vi "ACT_effective_setpoint.vi"(8 "error in (no error)":errorcluster, 11 "MD420 in":refnum<class "MD420.lvclass">) -> (0 "error out":errorcluster, 3 "MD420 out":refnum<class "MD420.lvclass">)   [LabVIEW 2022 SP3, in "MD420.lvclass"]
uses:
  MD420.lvclass
  SI_modules/SI656/SI656.lvclass
  SI_modules/SI657/SI657.lvclass
  MD420.lvclass/MD420.ctl
panel:
  in  "SI657.lvclass":refnum<class "SI657.lvclass">
  in  "SI656 in":refnum<class "SI656.lvclass">
  in  "PG SP-Grad":dbl
  in  "ACT-Ctrl ON (MD404)":dbl
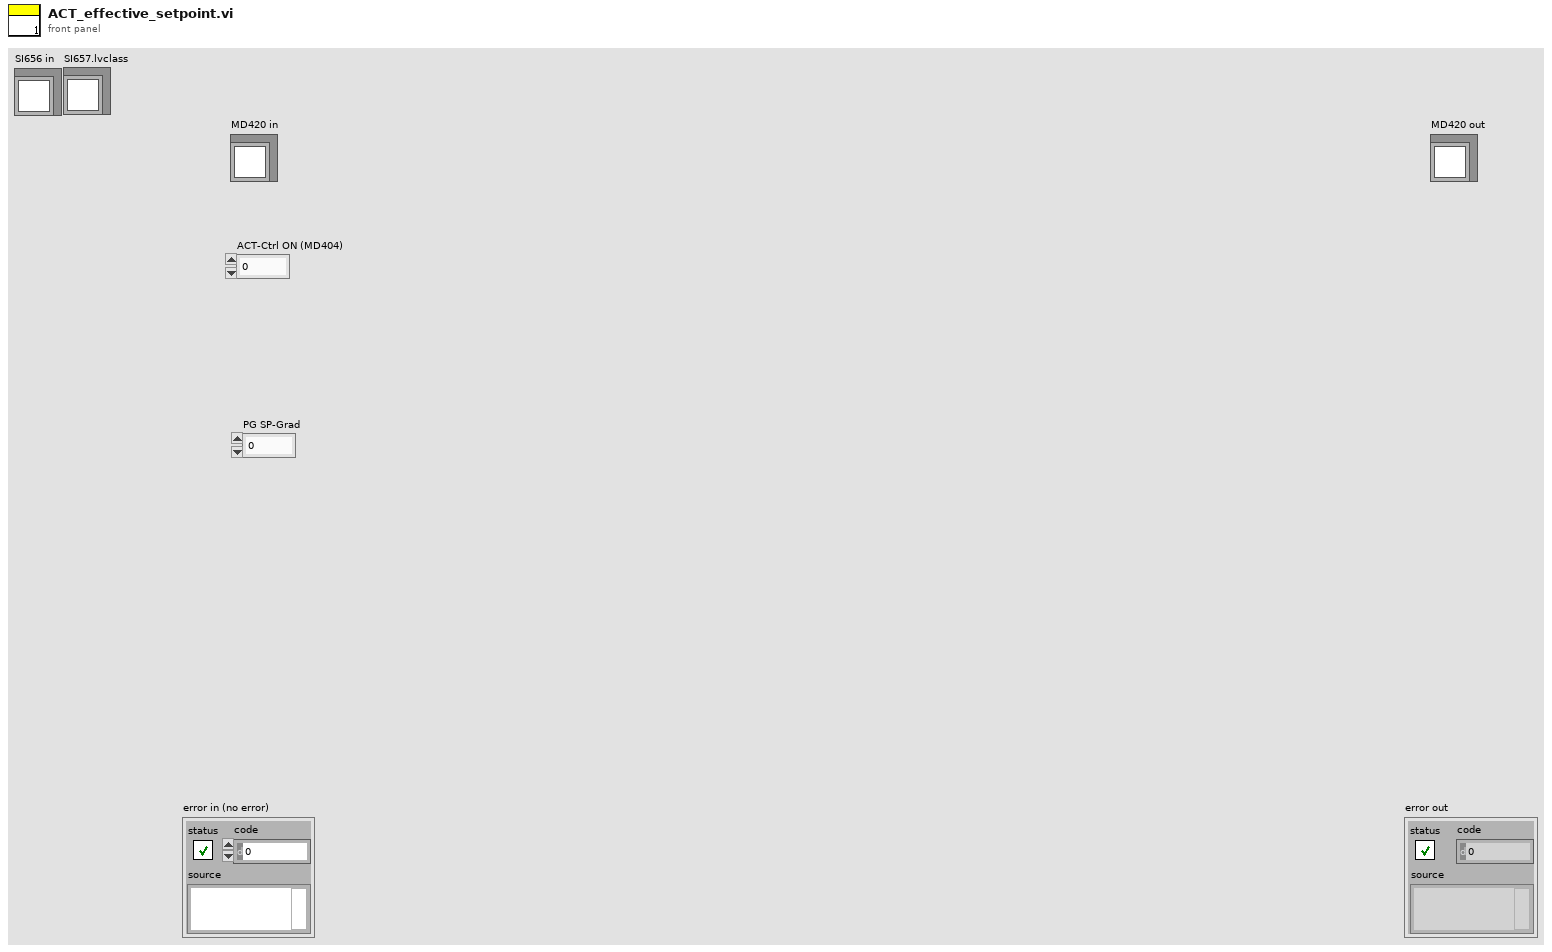
[diagram p1: front panel]
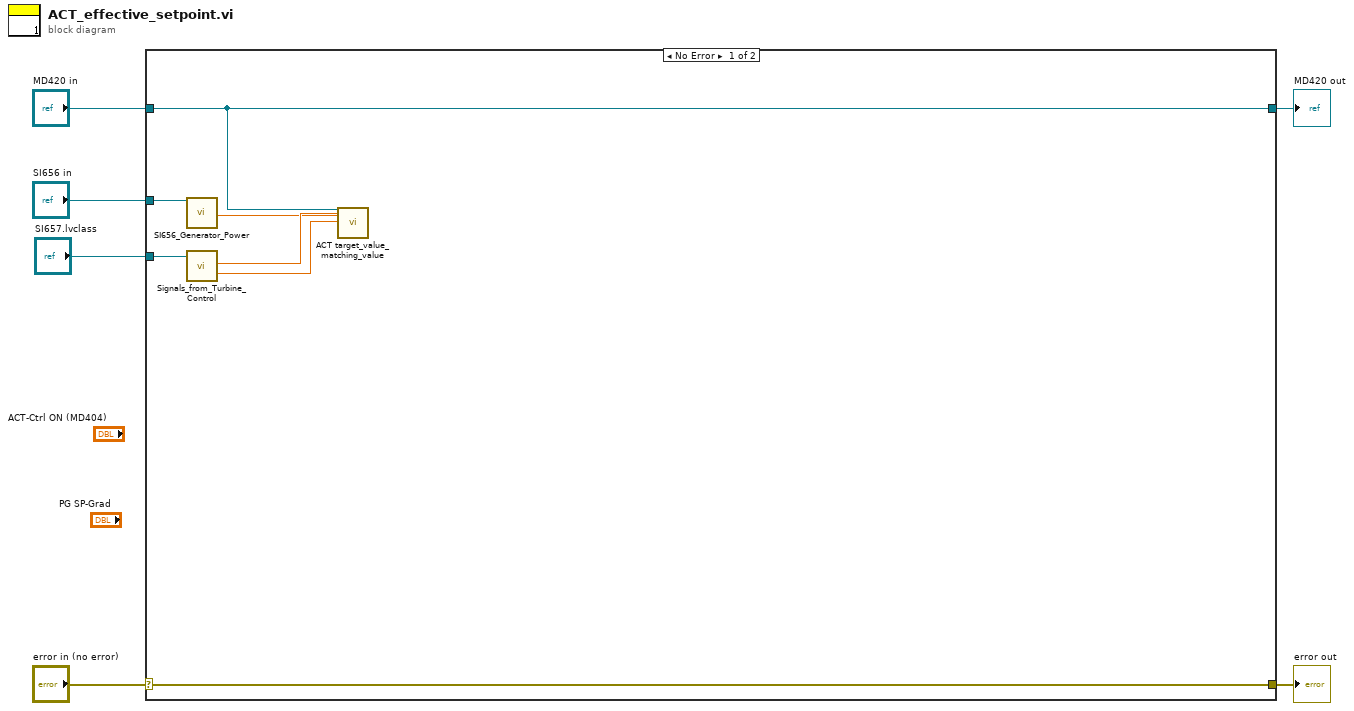
[diagram p0: block diagram]
diagram:
  n1 = case shown="No Error" "error in (no error)" {
    selector: "error in (no error)" -> [w13 w15]
    tunnel: [w13 w15] -> w5
    tunnel: [w11 w14] -> w3
    tunnel: "MD420 in" -> [w11 w14]
    tunnel: "SI656 in" -> [w10 _]
    tunnel: "SI657.lvclass" -> [w9 _]
    frame No Error {
      n2 = call "SI656_Generator_Power.vi"("SI656 in"=w10) -> ("PG 2nd Min in %"=w8:dbl)  [unwired: 15 in, 3 out]
      n3 = call "Signals_from_Turbine_Control.vi"("SI657.lvclass"=w9) -> ("PG eff SP"=w12:dbl, "PG target SP"=w7:dbl)  [unwired: 12 in, 5 out]
      n4 = call "ACT target_value_matching_value.vi"("MD420.lvclass"=w11, "PG eff SP"=w12, "PG 2nd Min in %"=w8, "PG target SP"=w7) -> ()  [unwired: 20 in, 4 out]
    }
    frame Error {
    }
  }
  "error out" <- w5
  "MD420 out" <- w3
